vi "Unregister for Sequence State Change Event.vi"(8 "error in (no error)":errorcluster, 11 "Sequence State Change Event Ref":T1) -> (0 "error out":errorcluster)   [LabVIEW 2020, in "NI_VS Sequence Execution Interface.lvlib"]
doc: "Unregisters a sequence state change event. Use the Register for Sequence State Change Event VI to get the <B>Sequence State Change Event Ref</B> this VI expects."
uses:
  <vilib>/NI VeriStand/Execution/SequenceExecutionInterface/NI_VS Sequence Execution Interface.lvlib
  <vilib>/NI VeriStand/Execution/SequenceExecutionInterface/Sequence State Change Event Ref.ctl
  <vilib>/NI VeriStand/Execution/SequenceExecutionInterface/Sequence State Change Event Data.ctl
  <vilib>/NI VeriStand/Execution/SequenceExecutionInterface/Sequence Execution State.ctl
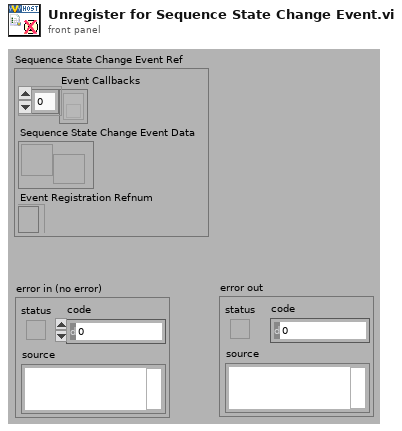
[diagram p1: front panel]
types:
  T1 = typedef "NI_VS Sequence Execution Interface.lvlib/Sequence State Change Event Ref.ctl" = cluster{"Event Callbacks":refnum<k27>[], "Sequence State Change Event Data":refnum<user-event>, "Event Registration Refnum":refnum<event-registration>}
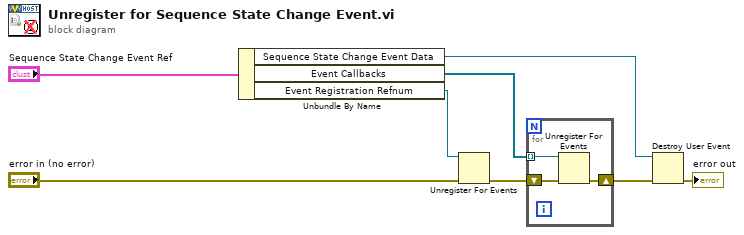
[diagram p0: block diagram]
diagram:
  n1 = Unbundle By Name("Sequence State Change Event Ref") -> ("Sequence State Change Event Data"=w2:refnum<user-event>, "Event Callbacks"=w5:refnum<k27>[], "Event Registration Refnum"=w7:refnum<event-registration>)
  n2 = Unregister For Events(event registration refnum=w7, error in="error in (no error)") -> (error out=w4:errorcluster)
  n3 = for {
    tunnel: w5 -> [w11] mode=indexing
    shift-right: [w9] -> w3
    shift-left: w4 -> [w10]
    n4 = Unregister For Events(event registration refnum=w11, error in=w10) -> (error out=w9:errorcluster)
  }
  n5 = Destroy User Event(user event=w2, error in=w3) -> (error out=→"error out":errorcluster)
